vi "log_line.vi"(10 "string":string, 11 "msg":refnum<vi>) -> ()   [LabVIEW 2016, in "MotionControl.lvlib"]
uses:
  <userlib>/MotionControl/MotionControl.lvlib
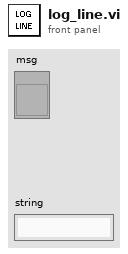
[diagram p1: front panel]
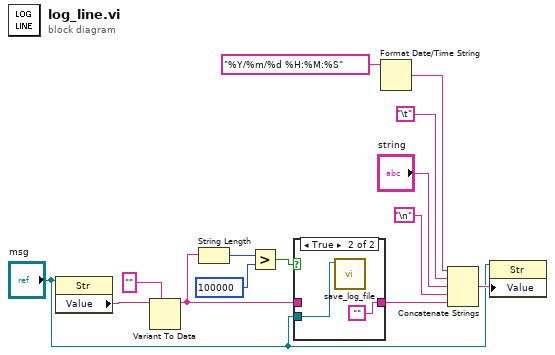
[diagram p0: block diagram]
diagram:
  n1 = property class="Str"(reference="msg") -> ("Value"=w9:string)  [unwired: 1 in, 2 out]
  n2 = Variant To Data(type="", Variant=w9) -> (data=w2:string)  [unwired: 1 in, 1 out]
  n3 = String Length(string=w2) -> (length=w6:i32)
  n4 = Greater?(x=w6, y=100000) -> (0:w4:bool)
  n5 = case shown="True" w4 {
    tunnel: "msg" -> [_ w17]
    tunnel: [w15 ""] -> w1
    tunnel: w2 -> [w15 _]
    frame False {
    }
    frame True {
      n6 = call <userlib>:"save_log_file.vi"("msg"=w17) -> ()  [unwired: 11 in]
    }
  }
  n7 = Format Date/Time String(time format string (%c)="%Y/%m/%d %H:%M:%S" ("时间格式字符串(%c)")) -> (date/time string=w10:string)  [unwired: 2 in]
  n8 = Concatenate Strings(w10, "\t", "string", "\n", w1) -> (w14:string)
  n9 = property class="Str"(reference="msg", "Value"=w14) -> ()  [unwired: 1 in, 2 out]
